vi "Error Cluster.Set VI Source.vi"(8 "class name (\"\")":string, 9 "library name (\"\")":string, 10 "vi name":string, 11 "error in":errorcluster) -> (1 "new offset":i32, 3 "error out":errorcluster)   [LabVIEW 2017, in "Memory Manager.lvlib" / "Static Error Handling.lvlib"]
doc: "Sets the error source VI of <b>error in</b>."
uses:
  Static Error Handling.lvlib
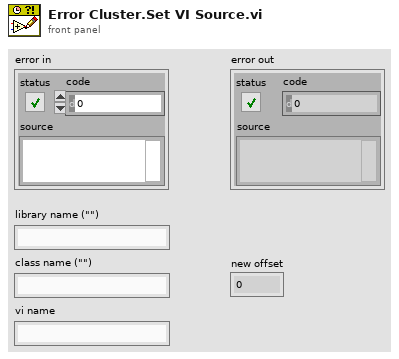
[diagram p1: front panel]
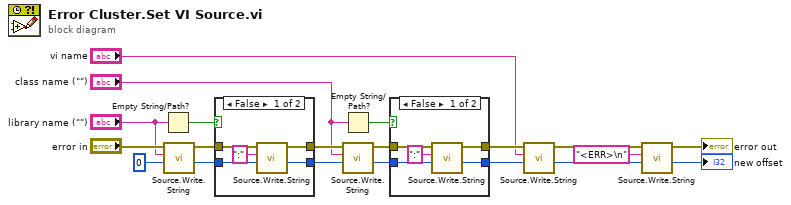
[diagram p0: block diagram]
diagram:
  n1 = Empty String/Path?(string/path="library name (\"\")") -> (empty?=w14:bool)
  n2 = call "Source.Write.String.vi"("offset"=0, "string"="library name (\"\")", "error in"="error in") -> ("new offset"=w12:i32, "error out"=w13:errorcluster)  [unwired: 7 in]
  n3 = case shown="False" w14 {
    tunnel: w13 -> [w25 w27]
    tunnel: w12 -> [w24 w26]
    tunnel: [w23 w27] -> w5
    tunnel: [w22 w26] -> w6
    frame False {
      n4 = call "Source.Write.String.vi"("offset"=w24, "string"=":", "error in"=w25) -> ("new offset"=w22:i32, "error out"=w23:errorcluster)  [unwired: 7 in]
    }
    frame True {
    }
  }
  n5 = Empty String/Path?(string/path="class name (\"\")") -> (empty?=w2:bool)
  n6 = call "Source.Write.String.vi"("offset"=w6, "string"="class name (\"\")", "error in"=w5) -> ("new offset"=w3:i32, "error out"=w4:errorcluster)  [unwired: 7 in]
  n7 = case shown="False" w2 {
    tunnel: w4 -> [w32 w34]
    tunnel: w3 -> [w31 w33]
    tunnel: [w30 w34] -> w9
    tunnel: [w29 w33] -> w8
    frame False {
      n8 = call "Source.Write.String.vi"("offset"=w31, "string"=":", "error in"=w32) -> ("new offset"=w29:i32, "error out"=w30:errorcluster)  [unwired: 7 in]
    }
    frame True {
    }
  }
  n9 = call "Source.Write.String.vi"("offset"=w8, "string"="vi name", "error in"=w9) -> ("new offset"=w11:i32, "error out"=w16:errorcluster)  [unwired: 7 in]
  n10 = call "Source.Write.String.vi"("offset"=w11, "string"="<ERR>\n", "error in"=w16) -> ("new offset"=→"new offset":i32, "error out"=→"error out":errorcluster)  [unwired: 7 in]
